vi "dfd_MRate G Check File Existence.vi"(6 "confirm?":bool=TRUE, 7 "# channels":i32=1, 8 "error in (no error)":errorcluster, 9 "filter name":string, 10 "dest path":path, 11 "multirate filters":T1[](array[typedef]) {"mMRate_SumWl" min=1 max=32 step=1; "mMRate_InputIwl" min=1 max=32 step=1; "mMRate_GainWl" min=1 max=32 step=1; "mMRate_OutputWl" min=1 max=32 step=1; "mMRate_InputWl" min=1 max=32 step=1; "mMRate_CoefWl" min=1 max=32 step=1; "mMRate_Mode" items=["Default"=-1, "No Rate Change"=0, "Interpolation"=1, "Decimation"=2, "Interpolated"=3, "Rational"=4]}) -> (0 "error out":errorcluster, 1 "filter name out":string)   [LabVIEW 2017, in "NI_DigFilterLicensed.lvlib"]
uses:
  <vilib>/addons/Digital Filter Design/NI_DigFilterLicensed.lvlib
  <vilib>/addons/Digital Filter Design/_Objects.llb/DFD Multirate Filter Obj.ctl
  <vilib>/addons/Digital Filter Design/_Objects.llb/DFD Multirate Mode.ctl
  <vilib>/addons/Digital Filter Design/_Objects.llb/DFD Coef Norm Type.ctl
  <vilib>/addons/Digital Filter Design/_Objects.llb/DFD Round-off Mode.ctl
  <vilib>/addons/Digital Filter Design/_Objects.llb/DFD FXP MRate Multiply Mode.ctl
  <vilib>/addons/Digital Filter Design/_Misc.llb/dfd_Error Handlers (Single).vi
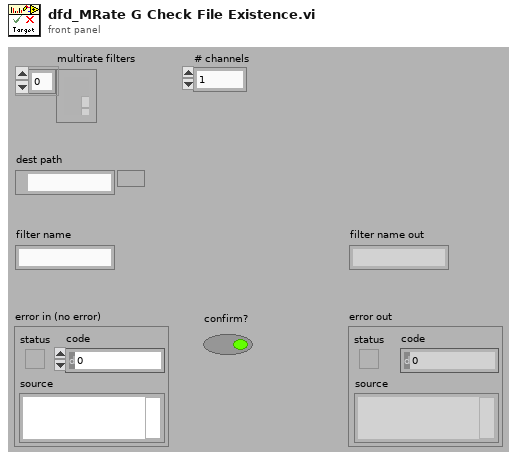
[diagram p1: front panel]
types:
  T1 = typedef "NI_DigFilterLicensed.lvlib/DFD Multirate Filter Obj.ctl" = cluster{"mMRate_Structure":enum16{"CIC", "FIR", "IIR", "Lattice"}, "mMRate_Mode":T2, "mMRate_Factor":i32, "mMRate_FIRParams":cluster{"mMRate_FIR_H":dbl[], "mMRate_FIR_IsNyquist?":bool, "mMRate_FIR_IsSymmetric?":bool}, "mMRate_CICParams":cluster{"mMRate_CIC_#Stage":i32, "mMRate_CIC_Lag":i32, "mMRate_CIC_Type":enum16{"Lowpass", "Highpass"}}, "mMRate_Order":i32, "mMRate_Version":string, "mMRate_Comments":string, "mMRate_RationalFactor":cluster{"mMRate_L":i32, "mMRate_M":i32}, "mMRate_Fs":dbl, "mMRate_Quantized?":bool, "mMRate_QFilterGain":dbl, "mMRate_CoefWl":i16, "mMRate_Scaling":cluster{"mMRate_ScaleByPowerOf2?":bool, "mMRate_ScaleType":T3}, "mMRate_InputWl":i16, "mMRate_OutputWl":i16, "mMRate_OutputMode":T4, "mMRate_MultMode":T5, "mMRate_BitPruning":bool, "mMRate_GainWl":i16, "mMRate_OutputFwl":i16, "mMRate_SumIwl":i16, "mMRate_InputIwl ":i16, "mMRate_SumWl":i16, "mMRate_CoefIwl":i16}
  T2 = typedef "NI_DigFilterLicensed.lvlib/DFD Multirate Mode.ctl" = i16
  T3 = typedef "NI_DigFilterLicensed.lvlib/DFD Coef Norm Type.ctl" = enum16{"No Norm", "Time Domain 1-Norm", "Time Domain 2-Norm", "Time Domain Inf-Norm"}
  T4 = typedef "NI_DigFilterLicensed.lvlib/DFD Round-off Mode.ctl" = enum16{"Nearest", "Truncation"}
  T5 = typedef "NI_DigFilterLicensed.lvlib/DFD FXP MRate Multiply Mode.ctl" = enum16{"Truncated", "Full"}
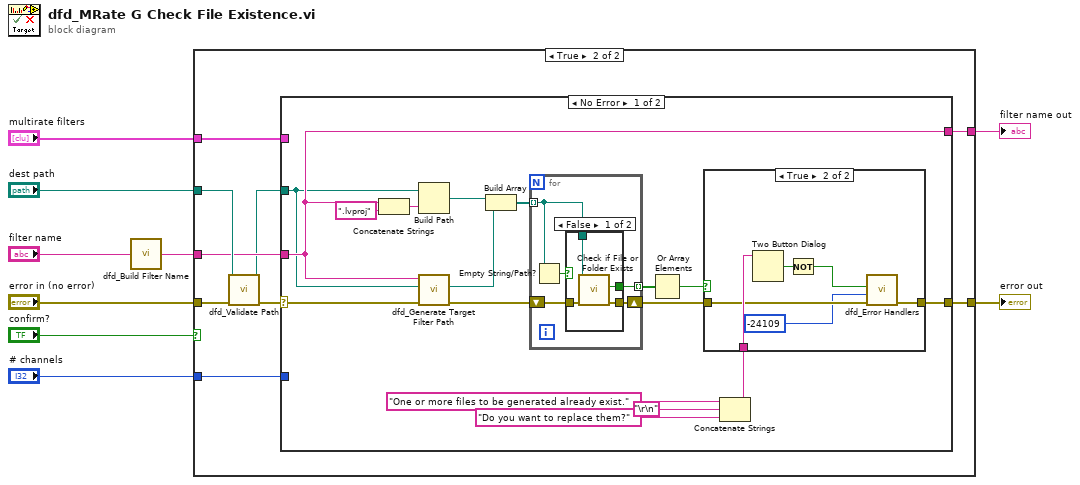
[diagram p0: block diagram]
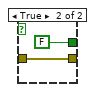
[diagram p4: hidden frame]
diagram:
  n1 = call <vilib>:"dfd_Build Filter Name.vi"("filter name in"="filter name") -> ("filter name out"=w1:string)
  n2 = case shown="True" "confirm?" {
    tunnel: "error in (no error)" -> [w10 w20]
    tunnel: "dest path" -> [_ w19]
    tunnel: w1 -> [w11 w18]
    tunnel: [w11 w16] -> w7
    tunnel: [w10 w14] -> w6
    tunnel: "multirate filters" -> [_ w13]
    tunnel: "# channels" -> [_ w12]
    frame False {
    }
    frame True {
      n3 = call <vilib>:"dfd_Validate Path.vi"("error in (no error)"=w20, "path in"=w19) -> ("error out"=w15:errorcluster, "path out"=w17:path)  [unwired: 8 out]
      n4 = case shown="No Error" w15 {
        selector: w15 -> [w35 w57]
        tunnel: w18 -> [w24 w56]
        tunnel: w17 -> [w21 _]
        tunnel: [w24 w56] -> w16
        tunnel: [w25 w57] -> w14
        tunnel: w13 -> [_ _]
        tunnel: w12 -> [_ _]
        frame No Error {
          n5 = Concatenate Strings(w24, ".lvproj" ("string")) -> (w36:string)
          n6 = Build Path(base path=w21, name or relative path=w36) -> (appended path=w22:path)
          n7 = call <vilib>:"dfd_Generate Target Filter Path.vi"("error in (no error)"=w35, "destination path"=w21, "filter name"=w24) -> ("error out"=w34:errorcluster, "target VI path"=w23:path)  [unwired: 7 out]
          n8 = Build Array(w22, w23) -> (w33:path[])
          n9 = for {
            tunnel: w33 -> [w46] mode=indexing
            shift-right: [w48] -> w30
            shift-left: w34 -> [w49]
            tunnel: [w47] -> w32 mode=indexing
            n10 = Empty String/Path?(string/path=w46) -> (empty?=w45:bool)
            n11 = case shown="False" w45 {
              tunnel: w49 -> [w53 w54]
              tunnel: w46 -> [w52 _]
              tunnel: [w51 w54] -> w48
              tunnel: [w50 FALSE ("file or folder exists?")] -> w47
              frame False {
                n12 = call <vilib>:"Check if File or Folder Exists.vi"("error in (no error)"=w53, "path"=w52) -> ("error out"=w51:errorcluster, "file or folder exists?"=w50:bool)  [unwired: 8 out]
              }
              frame True {
              }
            }
          }
          n13 = Or Array Elements(Boolean array=w32) -> (logical OR=w31:bool)
          n14 = Concatenate Strings("One or more files to be generated already exist.", "\r\n", "Do you want to replace them?") -> (w26:string)
          n15 = case shown="True" w31 {
            tunnel: w30 -> [w38 w43]
            tunnel: w26 -> [_ w44]
            tunnel: [w38 w42] -> w25
            frame False {
            }
            frame True {
              n16 = Two Button Dialog(message=w44) -> (T button?=w40:bool)  [unwired: 2 out]
              n17 = Not(x=w40) -> (.not. x?=w39:bool)
              n18 = call-poly <vilib>:"dfd_Error Handlers.vi"("error in (no error)"=w43, "error code"=-24109 ("ERR_CODEGEN_CANCELLED"), "condition failed?"=w39) -> ("error out"=w42:errorcluster)  [unwired: 8 out]
            }
          }
        }
        frame Error {
        }
      }
    }
  }
  "error out" <- w6
  "filter name out" <- w7
